vi "NI-DP__TransmitData.vi"(5 "Port to write to":u16=44515, 6 "timeout ms":u32=3000, 7 "IP to write to":string, 8 "error in":errorcluster, 10 "UDP-NI__Message":T1 {"Command" items=["0x01: Get Type & Hostname"=1, "0x03: Set IP 1"=3, "0x04: Set IP 2"=4, "0x08: Acknowledge"=8, "0x0A: Reboot"=10, "0x20: ???"=32, "0x21: ???"=33, "0xF2: System State"=242, "0xF4: System Details"=244]}, 11 "UDP Network Connection in":refnum<k16>) -> (0 "error out":errorcluster={"status"=TRUE, "code"=1, "source"="UDP Write in UDP-NI__SendData.vi"}, 3 "UDP Network Connection out":refnum<k16>)   [LabVIEW 2014, in "hse-network.lvlib"]
doc: "____\nHAMPEL SOFTWARE ENGINEERING v0.7.0 (2018-07-16 18:12)"
uses:
  hse-network.lvlib
  NI-DP__MessageStructure.ctl
  NI-DP__Commands.ctl
  hse-misc/hse-misc.lvlib
panel:
  out "resulting string":string
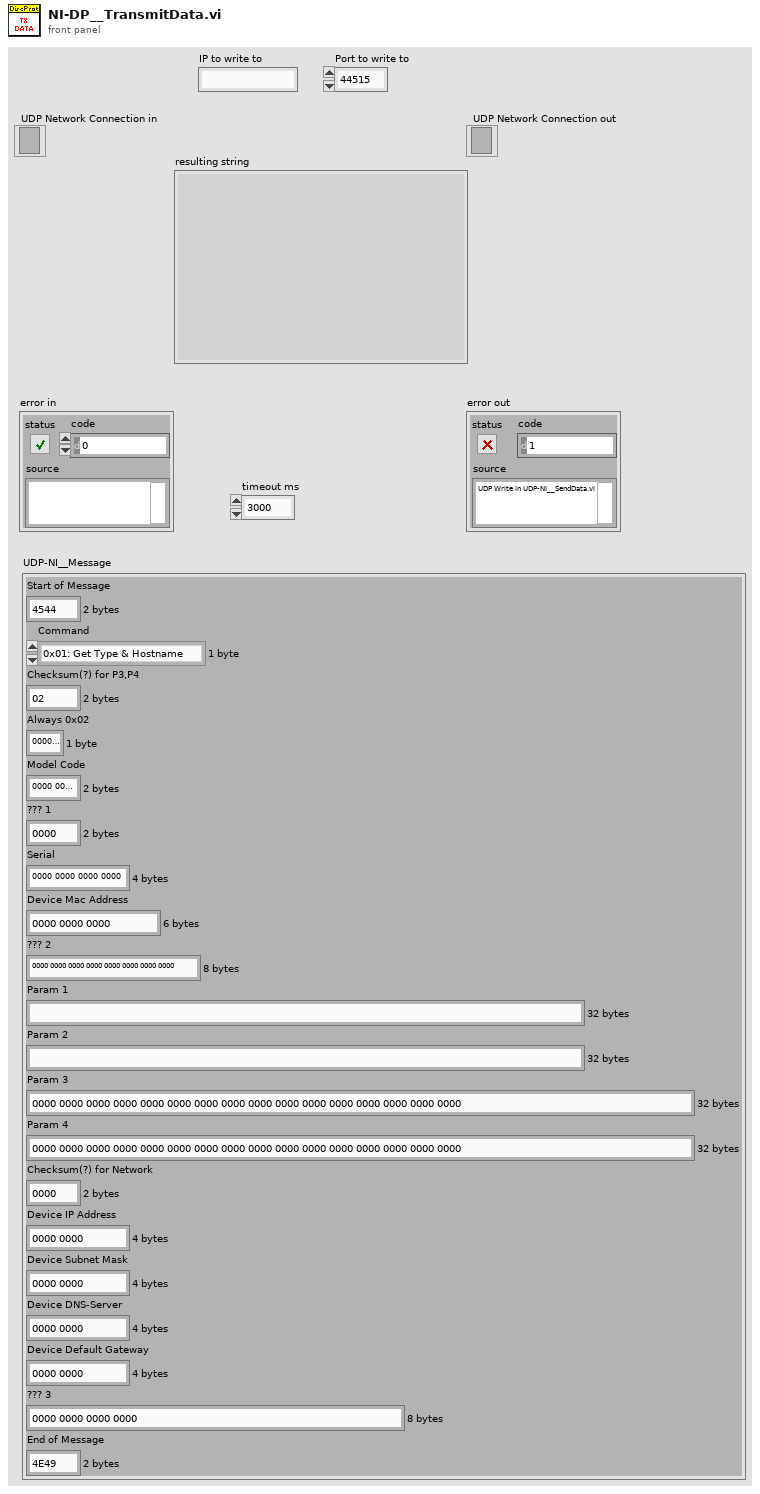
[diagram p1: front panel]
types:
  T1 = typedef "hse-network.lvlib/NI-DP__MessageStructure.ctl" = cluster{"Start of Message":string, "Command":T2, "Checksum(?) for P3,P4":string, "Always 0x02":string, "Model Code":string, "??? 1":string, "Serial":string, "Device Mac Address":string, "??? 2":string, "Param 1":string, "Param 2":string, "Param 3":string, "Param 4":string, "Checksum(?) for Network":string, "Device IP Address":string, "Device Subnet Mask":string, "Device DNS-Server":string, "Device Default Gateway":string, "??? 3":string, "End of Message":string}
  T2 = typedef "hse-network.lvlib/NI-DP__Commands.ctl" = u8
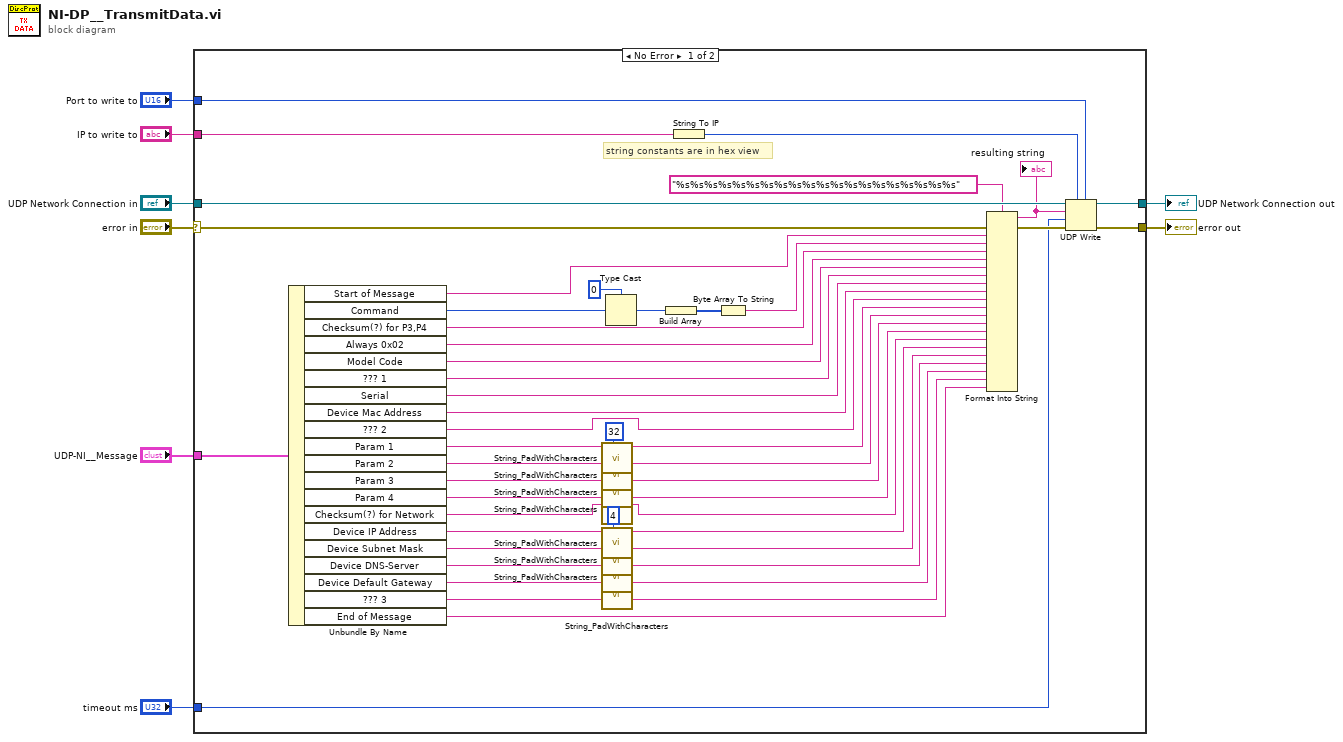
[diagram p0: block diagram]
diagram:
  n1 = case shown="No Error" "error in" {
    selector: "error in" -> [w48 w56]
    tunnel: [w54 w56] -> w8
    tunnel: "timeout ms" -> [w46 _]
    tunnel: [w53 w55] -> w6
    tunnel: "Port to write to" -> [w52 _]
    tunnel: "IP to write to" -> [w44 _]
    tunnel: "UDP Network Connection in" -> [w51 w55]
    tunnel: "UDP-NI__Message" -> [w40 _]
    frame No Error {
      w9 = 4 ("length")
      w28 = 32 ("length")
      # "string constants are in hex view"
      n2 = Unbundle By Name(w40) -> ("Start of Message"=w19:string, "Command"=w39:T2, "Checksum(?) for P3,P4"=w38:string, "Always 0x02"=w36:string, "Model Code"=w35:string, "??? 1"=w21:string, "Serial"=w20:string, "Device Mac Address"=w34:string, "??? 2"=w27:string, "Param 1"=w33:string, "Param 2"=w30:string, "Param 3"=w29:string, "Param 4"=w31:string, "Checksum(?) for Network"=w10:string, "Device IP Address"=w15:string, "Device Subnet Mask"=w16:string, "Device DNS-Server"=w17:string, "Device Default Gateway"=w18:string, "??? 3"=w23:string, "End of Message"=w22:string)
      n3 = call "String_PadWithCharacters.vi"("length"=w28, "str in"=w33) -> ("str (padded)"=w32:string)  [unwired: 9 in]
      n4 = call "String_PadWithCharacters.vi"("length"=w28, "str in"=w30) -> ("str (padded)"=w26:string)  [unwired: 9 in]
      n5 = call "String_PadWithCharacters.vi"("length"=w28, "str in"=w29) -> ("str (padded)"=w25:string)  [unwired: 9 in]
      n6 = call "String_PadWithCharacters.vi"("length"=w28, "str in"=w31) -> ("str (padded)"=w24:string)  [unwired: 9 in]
      n7 = call "String_PadWithCharacters.vi"("length"=w9, "str in"=w15) -> ("str (padded)"=w14:string)  [unwired: 9 in]
      n8 = call "String_PadWithCharacters.vi"("length"=w9, "str in"=w16) -> ("str (padded)"=w13:string)  [unwired: 9 in]
      n9 = call "String_PadWithCharacters.vi"("length"=w9, "str in"=w17) -> ("str (padded)"=w12:string)  [unwired: 9 in]
      n10 = call "String_PadWithCharacters.vi"("length"=w9, "str in"=w18) -> ("str (padded)"=w11:string)  [unwired: 9 in]
      n11 = Type Cast(type=u8 0, x=w39) -> (*(type *) &x=w41:u8)
      n12 = Build Array(w41) -> (w42:u8[])
      n13 = String To IP(1:w44) -> (0:w43:u32)
      n14 = Byte Array To String(unsigned byte array=w42) -> (string=w45:string)
      n15 = Format Into String(format string="%s%s%s%s%s%s%s%s%s%s%s%s%s%s%s%s%s%s%s%s", error in=w48, w19, w45, w38, w36, w35, w21, w20, w34, w27, w32, w26, w25, w24, w10, w14, w13, w12, w11, w23, w22) -> (resulting string=w49:string, error out=w47:errorcluster)  [unwired: 1 in]
      "resulting string" <- w49
      n16 = UDP Write(address=w43, port or service name=w52, connection ID=w51, data in=w49, 8:w47, 9:w46) -> (error out=w54:errorcluster, 3:w53:refnum<k16>)
    }
    frame Error {
    }
  }
  "error out" <- w8
  "UDP Network Connection out" <- w6
